vi "Cull and Group Boiler.vi"(6 "Line Border":cluster{"Top":dbl, "Bottom":dbl}={"Top"=6.0, "Bottom"=1.0}, 9 "Score Cutoff":dbl=3.0, 10 "Sorted Data":dbl[][](array[numeric])) -> (0 "Rect Out":T2 {"Bottom" format="%#_3g"; "Right" format="%#_3g"; "Top" format="%#_3g"; "Left" format="%#_3g"}, 1 "Line Out":T3, 2 "Score Out":dbl, 3 "Center Out":T1)   [LabVIEW 2017, in "VisionSystem.lvlib"]
doc: "Examine the particle measurements to find the most likely pair that make up the target. This mostly compares the edges of the bounding boxes. It then returns information about the overall target, notably the rectangle sourrounding the particles, the vertical line that bisects the target, and the center of the top particle."
uses:
  VisionSystem.lvlib
  Cluster_Line.ctl
  Cluster_UI DBL Box.ctl
  Cluster_SGL Point.ctl
panel:
  out "Grouping Scores":T4(array[cluster])
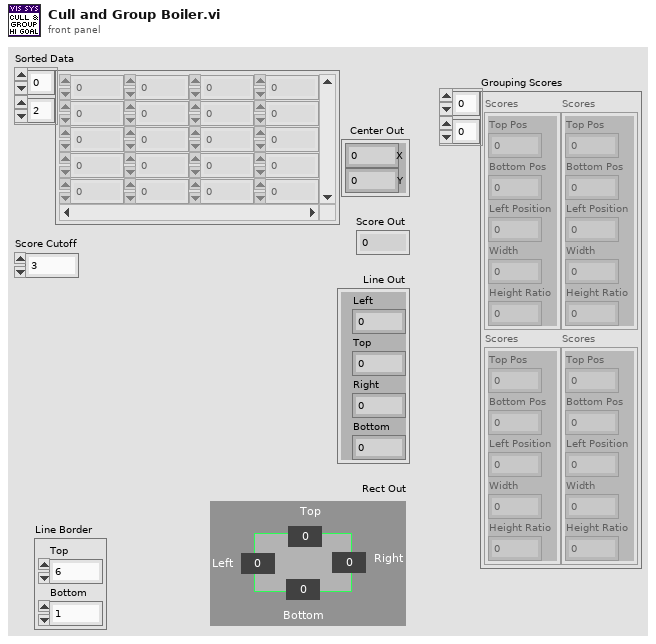
[diagram p1: front panel]
types:
  T1 = typedef "VisionSystem.lvlib/Cluster_SGL Point.ctl" = cluster{"X":sgl, "Y":sgl}
  T2 = typedef "VisionSystem.lvlib/Cluster_UI DBL Box.ctl" = cluster{"Left":dbl, "Top":dbl, "Right":dbl, "Bottom":dbl}
  T3 = typedef "VisionSystem.lvlib/Cluster_Line.ctl" = cluster{"Left":dbl, "Top":dbl, "Right":dbl, "Bottom":dbl}
  T4 = cluster{"Top Pos":dbl, "Bottom Pos":dbl, "Left Position":dbl, "Width":dbl, "Height Ratio":dbl}[][]
  T5 = typedef "Particle Parameters" = i32
  T6 = cluster{"Top Position":dbl, "Bottom Position":dbl, "Left Gap":dbl, "Width":dbl, "Height Ratio":dbl}
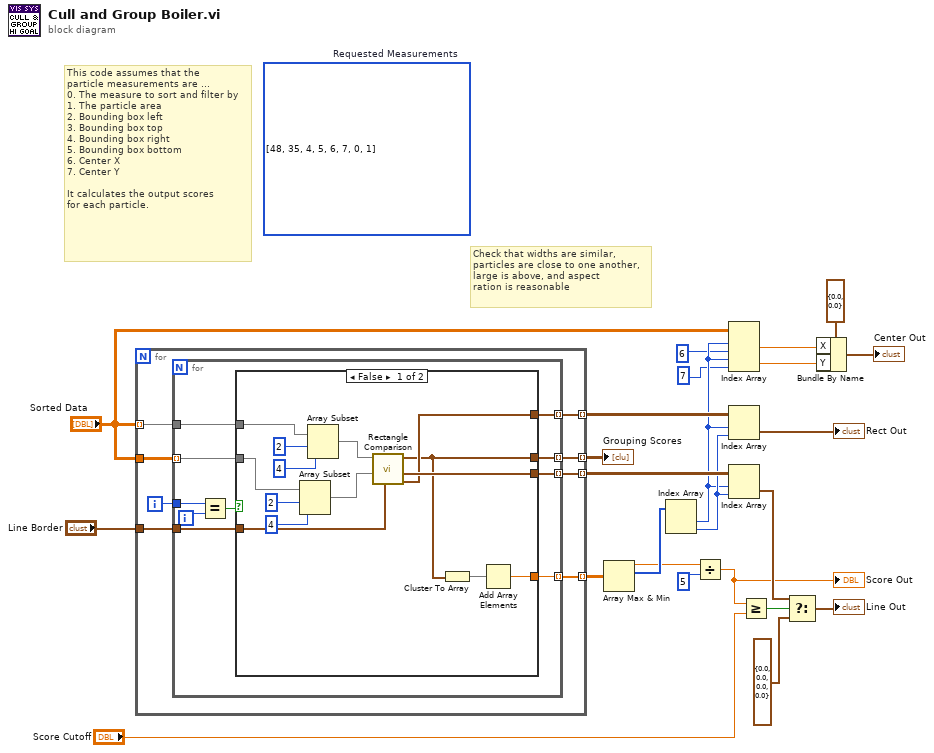
[diagram p0: block diagram]
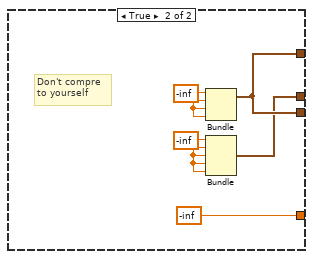
[diagram p2: hidden frame]
diagram:
  (unwired) T5[] [48, 35, 4, 5, 6, 7, 0, 1] items=["Center of Mass X", "Center of Mass Y", "First Pixel X", "First Pixel Y", "Bounding Rect Left", "Bounding Rect Top", "Bounding Rect Right", "Bounding Rect Bottom", "Max Feret Diameter Start X", "Max Feret Diameter Start Y", "Max Feret Diameter End X", "Max Feret Diameter End Y", "Max Horiz. Segment Length Left", "Max Horiz. Segment Length Right", "Max Horiz. Segment Length Row", "-", "Bounding Rect Width", "Bounding Rect Height", "Bounding Rect Diagonal", "Perimeter", "Convex Hull Perimeter", "Holes' Perimeter", "Max Feret Diameter", "Equivalent Ellipse Major Axis", "Equivalent Ellipse Minor Axis", "Equivalent Ellipse Minor Axis (Feret)", "Equivalent Rect Long Side", "Equivalent Rect Short Side", "Equivalent Rect Diagonal", "Equivalent Rect Short Side (Feret)", "Average Horiz. Segment Length", "Average Vert. Segment Length", "Hydraulic Radius", "Waddel Disk Diameter", "-", "Area", "Holes' Area", "Particle & Holes' Area", "Convex Hull Area", "Image Area", "-", "Number of Holes", "Number of Horiz. Segments", "Number of Vert. Segments", "-", "Orientation", "Max Feret Diameter Orientation", "-", "% Area/Image Area", "% Area/(Particle & Holes' Area)", "Ratio of Equivalent Ellipse Axes", "Ratio of Equivalent Rect Sides", "-", "Elongation Factor", "Compactness Factor", "Heywood Circularity Factor", "Type Factor", "-", "Sum X", "Sum Y", "Sum XX", "Sum XY", "Sum YY", "Sum XXX", "Sum XXY", "Sum XYY", "Sum YYY", "-", "Moment of Inertia XX", "Moment of Inertia XY", "Moment of Inertia YY", "Moment of Inertia XXX", "Moment of Inertia XXY", "Moment of Inertia XYY", "Moment of Inertia YYY", "Norm. Moment of Inertia XX", "Norm. Moment of Inertia XY", "Norm. Moment of Inertia YY", "Norm. Moment of Inertia XXX", "Norm. Moment of Inertia XXY", "Norm. Moment of Inertia XYY", "Norm. Moment of Inertia YYY", "Hu Moment 1", "Hu Moment 2", "Hu Moment 3", "Hu Moment 4", "Hu Moment 5", "Hu Moment 6", "Hu Moment 7"]  # Requested Measurements
  # "Check that widths are similar,\nparticles are close to one another,\nlarge is above, and aspect\nration is reasonable"
  # "This code assumes that the\nparticle measurements are ...\n0. The measure to sort and filter by\n1. The particle area\n2. Bounding box left\n3. Bounding box top\n4. Bounding box right\n5. Bounding box bottom\n6. Center X\n7. Center Y\n\nIt calculates the output scores\nfor each particle."
  n1 = for {
    tunnel: "Sorted Data" -> [w32] mode=indexing
    tunnel: "Sorted Data" -> [w31]
    tunnel: [w30] -> w24 mode=indexing
    tunnel: [w28] -> w23 mode=indexing
    tunnel: [w27] -> w20 mode=indexing
    tunnel: [w26] -> w16 mode=indexing
    tunnel: "Line Border" -> [w25]
    i -> [w29]
    n2 = for {
      tunnel: w32 -> [w42]
      tunnel: w31 -> [w40] mode=indexing
      tunnel: [w39] -> w30 mode=indexing
      tunnel: w29 -> [w38]
      tunnel: [w36] -> w28 mode=indexing
      tunnel: [w35] -> w27 mode=indexing
      tunnel: [w34] -> w26 mode=indexing
      tunnel: w25 -> [w33]
      i -> [w37]
      n3 = Equal?(x=w38, y=w37) -> (x = y?=w41:bool)
      n4 = case shown="False" w41 {
        tunnel: w42 -> [w54 _]
        tunnel: w40 -> [w51 _]
        tunnel: [w44 w57] -> w39
        tunnel: [w49 -inf] -> w36
        tunnel: [w46 w60] -> w35
        tunnel: [w45 w60] -> w34
        tunnel: w33 -> [w43 _]
        frame False {
          n5 = Array Subset(array=w51, index=2, length=4) -> (w47:dbl[])
          n6 = Array Subset(array=w54, index=2, length=4) -> (w48:dbl[])
          n7 = call "Rectangle Comparison.vi"("Line Border"=w43, "Second"=w47, "First"=w48) -> ("Rect Out"=w45:T2, "Line Out"=w46:T3, "Scores Out"=w44:T6)  [unwired: 6 in]
          n8 = Cluster To Array(cluster=w44) -> (array=w50:dbl[])
          n9 = Add Array Elements(numeric array=w50) -> (sum=w49:dbl)
        }
        frame True {
          w58 = -inf
          w59 = -inf
          # "Don't compre\nto yourself"
          n10 = Bundle(w59, w59, w59, w59) -> (w60:cluster{dbl, dbl, dbl, dbl})  [unwired: 1 in]
          n11 = Bundle(w58, w58, w58, w58, w58) -> (w57:cluster{dbl, dbl, dbl, dbl, dbl})  [unwired: 1 in]
        }
      }
    }
  }
  "Grouping Scores" <- w24
  n12 = Array Max & Min(array=w23) -> (max value=w5:dbl, max index (indices)=w6:i32[])  [unwired: 2 out]
  n13 = Index Array(array=w6) -> (element #1=w12:i32, element #2=w15:i32)  [unwired: 2 in]
  n14 = Divide(x=w5, y=5 ("length")) -> (x/y=w4:dbl)
  "Score Out" <- w4
  n15 = Index Array(array="Sorted Data", index (row) #1=w12, index (col) #1=6 ("index"), index (row) #2=w12, index (col) #2=7 ("index")) -> (element #1=w10:dbl, element #2=w9:dbl)
  n16 = Index Array(array=w16, index (row)=w12, index (col)=w15) -> (element=→"Rect Out":T2)
  n17 = Index Array(array=w20, index (row)=w12, index (col)=w15) -> (element=w19:T3)
  n18 = Greater Or Equal?(x=w4, y="Score Cutoff") -> (x >= y?=w22:bool)
  n19 = Select(t=w19, s=w22, f=T3 {"Left"=0.0, "Top"=0.0, "Right"=0.0, "Bottom"=0.0}) -> (s? t:f=→"Line Out":T3)
  n20 = Bundle By Name(cluster=T1 {"X"=0.0, "Y"=0.0} ("Center Out"), "X"=w10, "Y"=w9) -> (→"Center Out":T1)
